vi "RegisterImagePixelPtr.vi"(8 "error in":errorcluster, 9 "Y Coordinate":i32, 10 "X Coordinate":i32, 11 "Image Reference In":T2) -> (0 "error out":errorcluster, 2 "PixelPointer":T1 {"Pixel Pointer" format="%.0x"}, 3 "Image Reference Out":T2)   [LabVIEW 2020, in "OpenLvVision_Image.lvlib" / "DataAccess.lvlib"]
doc: "Returns the pixel memory pointer and alignment details."
uses:
  DataAccess.lvlib
  Management/TypeDef/Image.ctl
  TypeDef/PixelPointer.ctl
  Management/Management.lvlib
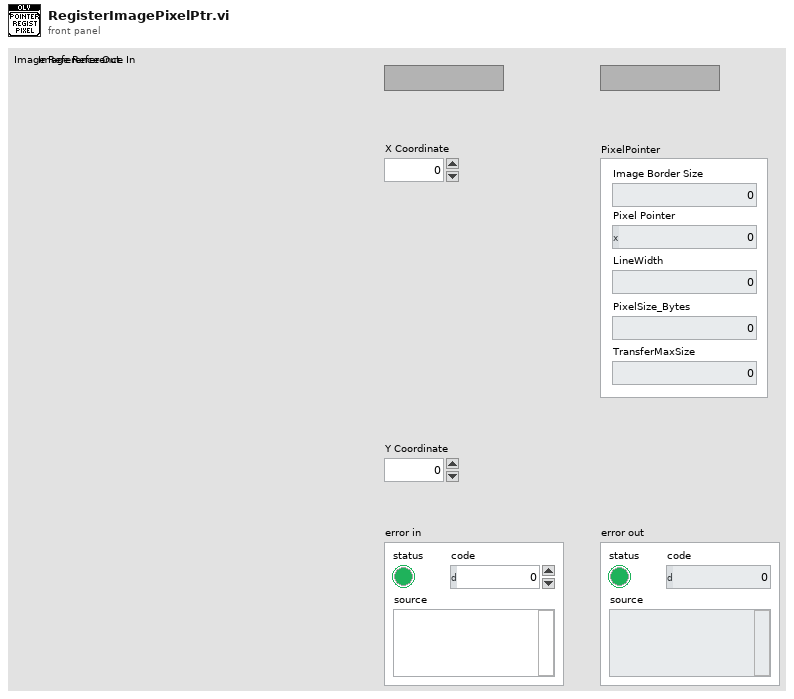
[diagram p1: front panel]
types:
  T1 = typedef "OpenLvVision_Image.lvlib/DataAccess.lvlib/PixelPointer.ctl" = cluster{"Image Border Size":i32, "Pixel Pointer":u64, "LineWidth":i32, "PixelSize_Bytes":i32, "TransferMaxSize":i32}
  T2 = typedef "OpenLvVision_Image.lvlib/Management.lvlib/Image.ctl" = refnum<image>
  T3 = enum32{"Map Pixel Pointer", "Unmap Pixel Pointer", "Get Pixels Infos"}
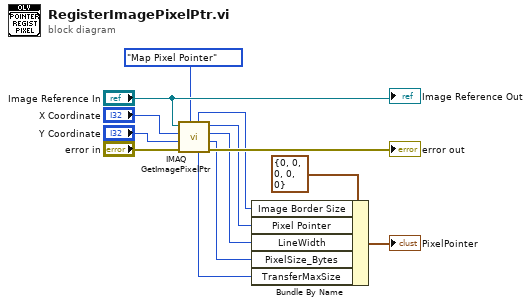
[diagram p0: block diagram]
diagram:
  n1 = call "IMAQ GetImagePixelPtr"("Function"=T3."Map Pixel Pointer", "error in (no error)"="error in", "Y Coordinate"="Y Coordinate", "X Coordinate"="X Coordinate", "Image"="Image Reference In") -> ("error out"=→"error out":errorcluster, "Pixel Size (Bytes)"=w2:i32, "LineWidth(Pixels)"=w3:i32, "Pixel Pointer out"=w4:u64, "Transfer Max Size"=w1:i32, "Image Border Size"=w8:i32)  [unwired: 1 in]
  n2 = Bundle By Name(cluster=T1 {"Image Border Size"=0, "Pixel Pointer"=0, "LineWidth"=0, "PixelSize_Bytes"=0, "TransferMaxSize"=0} ("PixelPointer"), "Image Border Size"=w8, "Pixel Pointer"=w4, "LineWidth"=w3, "PixelSize_Bytes"=w2, "TransferMaxSize"=w1) -> (→"PixelPointer":T1)
  "Image Reference Out" <- "Image Reference In"
